vi "Global Mapper A.vi"(11 "GIC Input":T1={"     Use ?\nOff       On"=[FALSE, TRUE, FALSE, TRUE], "Mode:"=FALSE, "WP Data"="", "Hokuyo Port"="COM7", "Prop  Port"="COM6", "Compass Port"="", "GPS Port"="", "Num of WPs"=0, "WP Lats and Longs"={"WP Lats"=[], "WP Longs"=[]}, "Obst Lats and Longs"={"Obst Lats"=[], "Obst Longs"=[]}, "Parameters"=[], "GPS Data"=[], "Compass"=0.0, "LMS Vector"=[], "Vision Vector"=[], "Direction Cmd"=0.0, "Speed Cmd"=0.0, "WP Vector"=[], "WP Number"=0, "Extra"=0, "SW Map"=[], "Path Cluster"={"Path x node"=[], "Path y node"=[]}} {"Obst Lats and Longs"."Obst Longs" format="%#_8g"; "Obst Lats and Longs"."Obst Lats" format="%#_8g"}) -> (3 "Robot and WPs":picture)   [LabVIEW 2014]
panel:
  # "Global Mapper A"
  # "Input:"
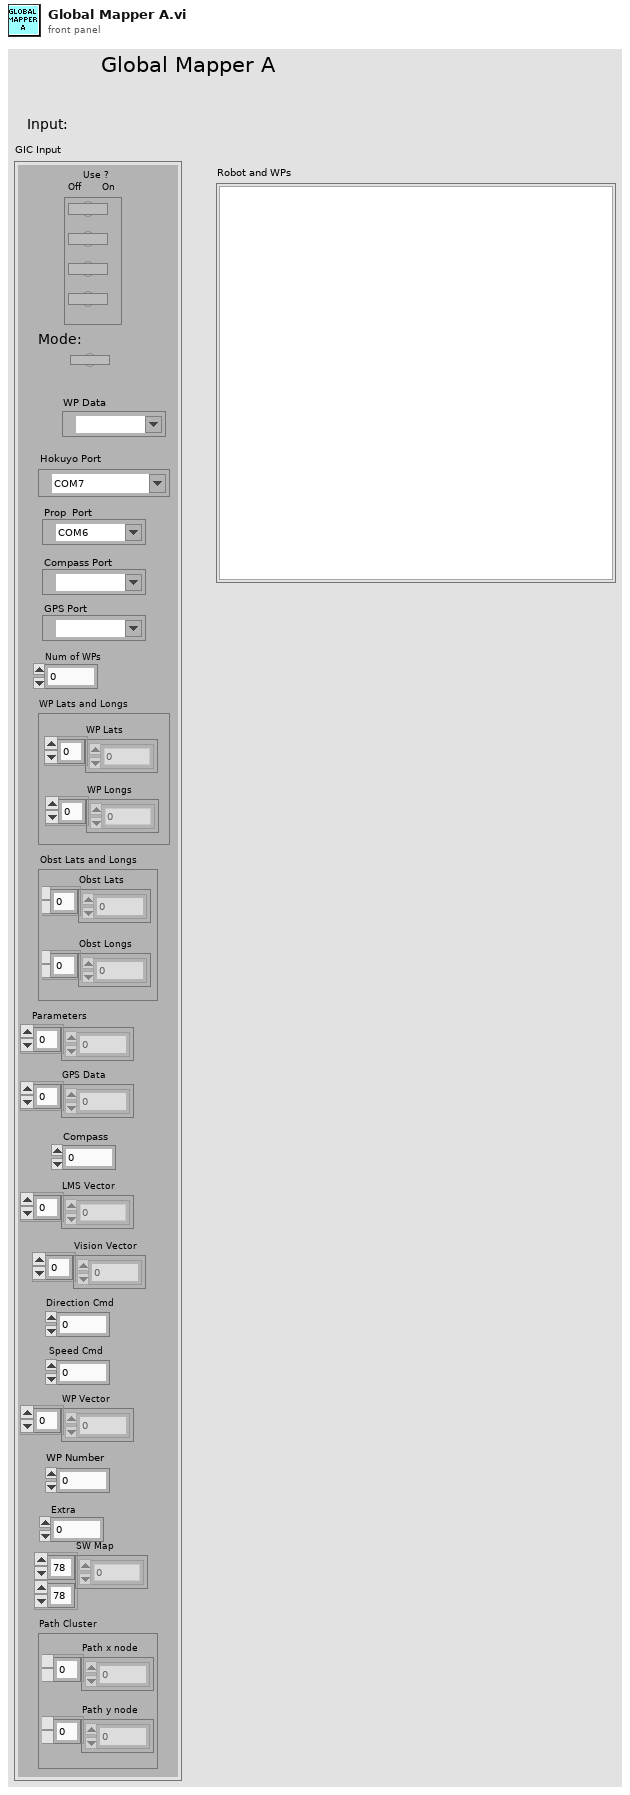
[diagram p1: front panel]
types:
  T1 = cluster{"     Use ?\nOff       On":bool[], "Mode:":bool, "WP Data":refnum<visa-resource-name>, "Hokuyo Port":refnum<visa-resource-name>, "Prop  Port":refnum<visa-resource-name>, "Compass Port":refnum<visa-resource-name>, "GPS Port":refnum<visa-resource-name>, "Num of WPs":i16, "WP Lats and Longs":cluster{"WP Lats":dbl[], "WP Longs":dbl[]}, "Obst Lats and Longs":cluster{"Obst Lats":dbl[], "Obst Longs":dbl[]}, "Parameters":dbl[], "GPS Data":dbl[], "Compass":dbl, "LMS Vector":dbl[], "Vision Vector":dbl[], "Direction Cmd":dbl, "Speed Cmd":dbl, "WP Vector":dbl[], "WP Number":i32, "Extra":i16, "SW Map":i32[][], "Path Cluster":cluster{"Path x node":dbl[], "Path y node":dbl[]}}
  T2 = cluster{"Width":u16, "Style":enum32{"Solid", "Dash", "Dot", "DashDot", "DashDotDot"}}
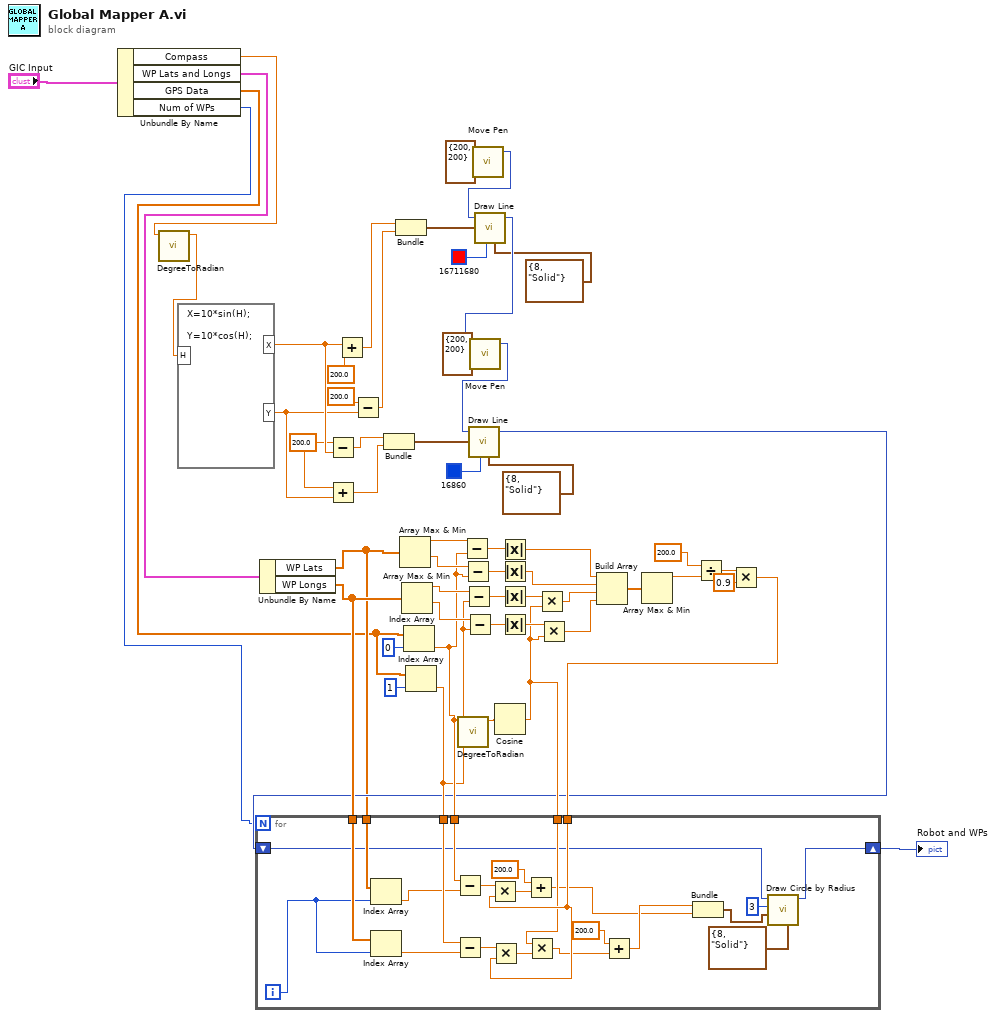
[diagram p0: block diagram]
diagram:
  w42 = 200.0 ("x")
  n1 = Unbundle By Name("GIC Input") -> ("Compass"=w5:dbl, "WP Lats and Longs"=w4:cluster{"WP Lats":dbl[], "WP Longs":dbl[]}, "GPS Data"=w3:dbl[], "Num of WPs"=w2:i16)
  n2 = call "DegreeToRadian.vi"("Degrees"=w5) -> ("Radians"=w38:dbl)  [unwired: 10 in]
  n3 = formula code="X=10*sin(H);\n\nY=10*cos(H);"("H"=w38) -> ("X"=w44:dbl, "Y"=w41:dbl)
  n4 = Unbundle By Name(w4) -> ("WP Lats"=w6:dbl[], "WP Longs"=w12:dbl[])
  n5 = Subtract(x=w42, y=w44) -> (x-y=w43:dbl)
  n6 = Add(x=w42, y=w41) -> (x+y=w40:dbl)
  n7 = Add(x=w44, y=200.0) -> (x+y=w48:dbl)
  n8 = Subtract(x=200.0, y=w41) -> (x-y=w46:dbl)
  n9 = Bundle(w43, w40) -> (w39:cluster{dbl, dbl})  [unwired: 1 in]
  n10 = Bundle(w48, w46) -> (w45:cluster{dbl, dbl})  [unwired: 1 in]
  n11 = Array Max & Min(array=w6) -> (max value=w33:dbl, min value=w18:dbl)  [unwired: 2 out]
  n12 = Array Max & Min(array=w12) -> (max value=w30:dbl, min value=w27:dbl)  [unwired: 2 out]
  n13 = Index Array(array=w3, index=0) -> (element=w13:dbl)
  n14 = Index Array(array=w3, index=1) -> (element=w11:dbl)
  n15 = call "DegreeToRadian.vi"("Degrees"=w13) -> ("Radians"=w16:dbl)  [unwired: 10 in]
  n16 = Subtract(x=w33, y=w13) -> (x-y=w32:dbl)
  n17 = Subtract(x=w18, y=w13) -> (x-y=w31:dbl)
  n18 = Subtract(x=w30, y=w11) -> (x-y=w29:dbl)
  n19 = Subtract(x=w27, y=w11) -> (x-y=w26:dbl)
  n20 = call <vilib>:"Move Pen.vi"("new position"=cluster{"x":i16, "y":i16} {"x"=200, "y"=200}) -> ("new picture"=w55:picture)  [unwired: 4 in]
  n21 = call <vilib>:"Draw Line.vi"("picture"=w55, "end point"=w45, "color(black)"=u32 16711680, "pen"=T2 {"Width"=8, "Style"=enum."Solid"}) -> ("new picture"=w53:picture)  [unwired: 5 in]
  n22 = call <vilib>:"Move Pen.vi"("new position"=cluster{"x":i16, "y":i16} {"x"=200, "y"=200}, "picture"=w53) -> ("new picture"=w51:picture)  [unwired: 3 in]
  n23 = call <vilib>:"Draw Line.vi"("picture"=w51, "end point"=w39, "color(black)"=u32 16860, "pen"=T2 {"Width"=8, "Style"=enum."Solid"}) -> ("new picture"=w7:picture)  [unwired: 5 in]
  n24 = Cosine(x=w16) -> (cos(x)=w9:dbl)
  n25 = Absolute Value(x=w32) -> (abs(x)=w20:dbl)
  n26 = Absolute Value(x=w31) -> (abs(x)=w19:dbl)
  n27 = Absolute Value(x=w29) -> (abs(x)=w28:dbl)
  n28 = Absolute Value(x=w26) -> (abs(x)=w25:dbl)
  n29 = Multiply(x=w28, y=w9) -> (x*y=w24:dbl)
  n30 = Multiply(x=w25, y=w9) -> (x*y=w23:dbl)
  n31 = Build Array(w20, w19, w24, w23) -> (w22:dbl[])
  n32 = Array Max & Min(array=w22) -> (max value=w17:dbl)  [unwired: 3 out]
  n33 = Divide(x=200.0, y=w17) -> (x/y=w15:dbl)
  n34 = Multiply(x=w15, y=0.9) -> (x*y=w10:dbl)
  n35 = for {
    N: w2 -> [_]
    tunnel: w13 -> [w79]
    tunnel: w12 -> [w62]
    tunnel: w11 -> [w75]
    tunnel: w10 -> [w73]
    tunnel: w9 -> [w70]
    shift-right: [w68] -> w8
    shift-left: w7 -> [w57]
    tunnel: w6 -> [w61]
    i -> [w58]
    n36 = Index Array(array=w61, index=w58) -> (element=w60:dbl)
    n37 = Index Array(array=w62, index=w58) -> (element=w59:dbl)
    n38 = Subtract(x=w79, y=w60) -> (x-y=w78:dbl)
    n39 = Subtract(x=w75, y=w59) -> (x-y=w74:dbl)
    n40 = Multiply(x=w78, y=w73) -> (x*y=w77:dbl)
    n41 = Multiply(x=w74, y=w73) -> (x*y=w71:dbl)
    n42 = Add(x=200.0, y=w77) -> (x+y=w63:dbl)
    n43 = Multiply(x=w70, y=w71) -> (x*y=w69:dbl)
    n44 = Add(x=200.0, y=w69) -> (x+y=w64:dbl)
    n45 = Bundle(w64, w63) -> (w66:cluster{dbl, dbl})  [unwired: 1 in]
    n46 = call <vilib>:"Draw Circle by Radius.vi"("pen"=T2 {"Width"=8, "Style"=enum."Solid"}, "pixel center"=w66, "radius"=i16 3, "picture"=w57) -> ("new picture"=w68:picture)  [unwired: 7 in]
  }
  "Robot and WPs" <- w8
